vi "LabVIEW TestStand Process Memory Usage.vi"() -> ()   [LabVIEW 2016]
panel:
  in  "Log File Folder Path (use dialog)":path=path "D:/log.csv"
  out "Sequence Editor Thread Count":u32
  out "Sequence Editor  HandleCount":u32
  out "Sequence Editor Memory (MB)":u64
  in  "interval (s)":dbl=3.0
  out "Memory Usage":cluster{"HandleCount":dbl, "HandleCount":dbl}(graph)
  out "LabVIEW Memory Used (MB)":u64
  out "LabVIEW Thread Count":u32
  out "error out":errorcluster
  out "LabVIEW HandleCount":u32
  in  "stop":bool
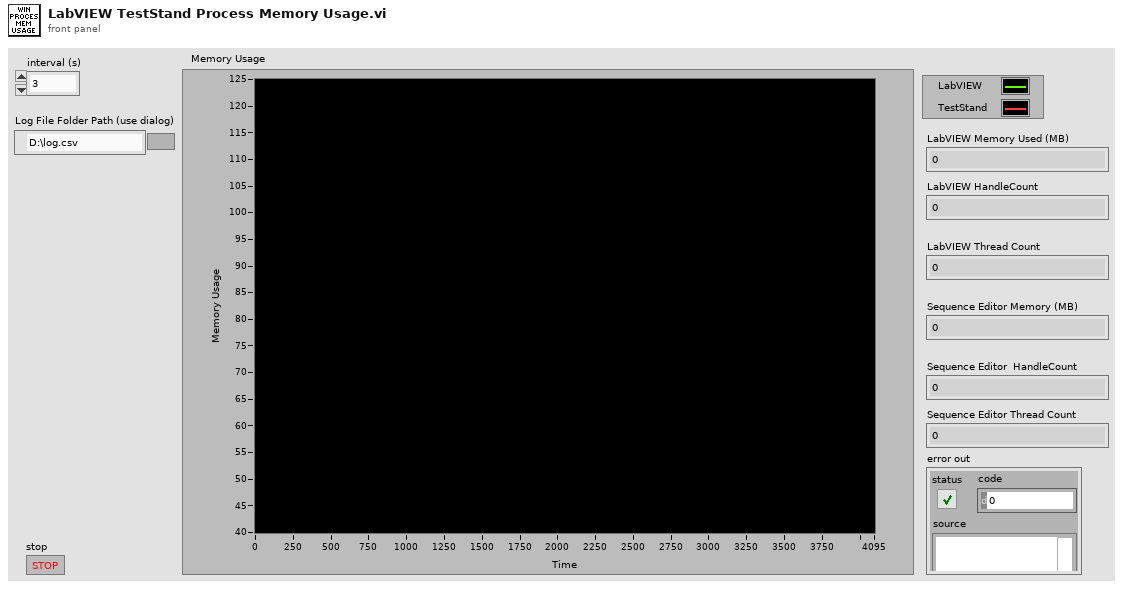
[diagram p1: front panel]
types:
  T1 = cluster{"LabVIEW  Memory Used (MB)":dbl, "Sequence Editor Memory (MB)":dbl}
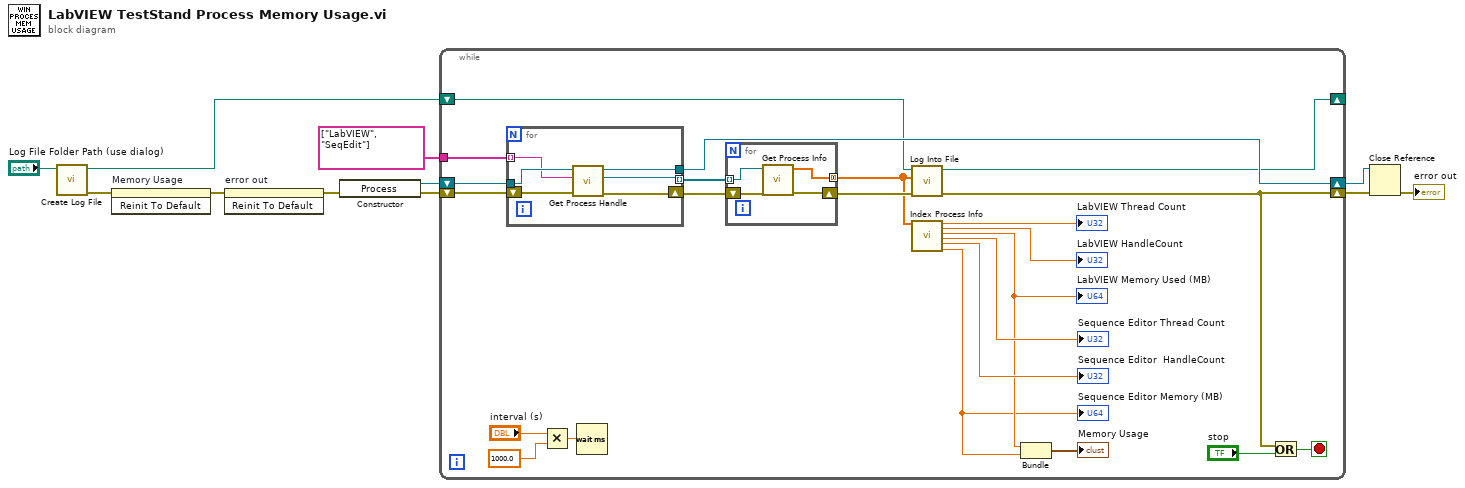
[diagram p0: block diagram]
diagram:
  n1 = call "Create Log File.vi"("File Path (use dialog)"="Log File Folder Path (use dialog)") -> ("error out"=w5:errorcluster, "log file path"=w4:path)  [unwired: 9 in]
  n2 = invoke on="Memory Usage" class="WFChart (strict)" method="Reinit To Default"(error in=w5) -> (error out=w2:errorcluster)  [unwired: 2 in, 2 out]
  n3 = invoke on="error out" class="Clust (strict)" method="Reinit To Default"(error in=w2) -> (error out=w1:errorcluster)  [unwired: 2 in, 2 out]
  n4 = constructor class="Process"(error in=w1) -> (reference out=w9:refnum<k24>, error out=w10:errorcluster)  [unwired: 2 in, 1 out]
  n5 = while {
    tunnel: string[] ["LabVIEW", "SeqEdit"] -> [w29]
    shift-right: [w20] -> w8
    shift-left: w10 -> [w30]
    shift-right: [w22] -> _
    shift-left: w4 -> [w23]
    shift-right: [w25] -> w7
    shift-left: w9 -> [w28]
    stop <- w21 stop-if-true
    n6 = for {
      tunnel: w29 -> [w41] mode=indexing
      tunnel: [w43] -> w25
      tunnel: w28 -> [w42]
      tunnel: [w40] -> w27 mode=indexing
      shift-right: [w39] -> w26
      shift-left: w30 -> [w44]
      n7 = call "Get Process Handle.vi"("error in (no error)"=w44, "processName"=w41, ".NET Refnum in"=w42) -> ("error out"=w39:errorcluster, "target process handle"=w40:refnum<k24>, ".NET Refnum out"=w43:refnum<k24>)  [unwired: 6 in]
    }
    n8 = Multiply(x="interval (s)", y=1000.0) -> (x*y=w33:dbl)
    n9 = Wait (ms)(milliseconds to wait=w33) -> ()  [unwired: 1 out]
    n10 = for {
      tunnel: w27 -> [w38] mode=indexing
      shift-right: [w36] -> w24
      shift-left: w26 -> [w37]
      tunnel: [w35] -> w12 mode=concatenating
      n11 = call "Get Process Info.vi"("error in (no error)"=w37, "process handle"=w38) -> ("error out"=w36:errorcluster, "process information"=w35:dbl[])  [unwired: 8 in]
    }
    n12 = call "Log Into File.vi"("error in"=w24, "Memory Information"=w12, "file path in"=w23) -> ("error out"=w20:errorcluster, "file path out"=w22:path)  [unwired: 7 in]
    n13 = call "Index Process Info.vi"("process information"=w12) -> ("LabVIEW Thread Count"=→"LabVIEW Thread Count":dbl, "LabVIEW HandleCount"=→"LabVIEW HandleCount":dbl, "LabVIEW  Memory Used (MB)"=w15:dbl, "Sequence Editor Thread Count"=→"Sequence Editor Thread Count":dbl, "Sequence Editor  HandleCount"=→"Sequence Editor  HandleCount":dbl, "Sequence Editor Memory (MB)"=w14:dbl)  [unwired: 13 in]
    "LabVIEW Memory Used (MB)" <- w15
    "Sequence Editor Memory (MB)" <- w14
    n14 = Bundle("LabVIEW  Memory Used (MB)"=w15, "Sequence Editor Memory (MB)"=w14) -> (→"Memory Usage":T1)  [unwired: 1 in]
    n15 = Or(x=w20, y="stop") -> (x .or. y?=w21:bool)
  }
  n16 = Close Reference(reference=w7, error in (no error)=w8) -> (error out=→"error out":errorcluster)
